vi "read_params.vi"(8 "error in (no error)":errorcluster, 11 "GaussianNB in":refnum<class "GaussianNB.lvclass">) -> (0 "error out":errorcluster, 2 "params":T1={"priors"=[], "var_smoothing"=1e-09}, 3 "GaussianNB out":refnum<class "GaussianNB.lvclass">)   [LabVIEW 2020, in "GaussianNB.lvclass"]
uses:
  GaussianNB.lvclass
  Controls/gaussian_nb_params.ctl
  GaussianNB.lvclass/GaussianNB.ctl
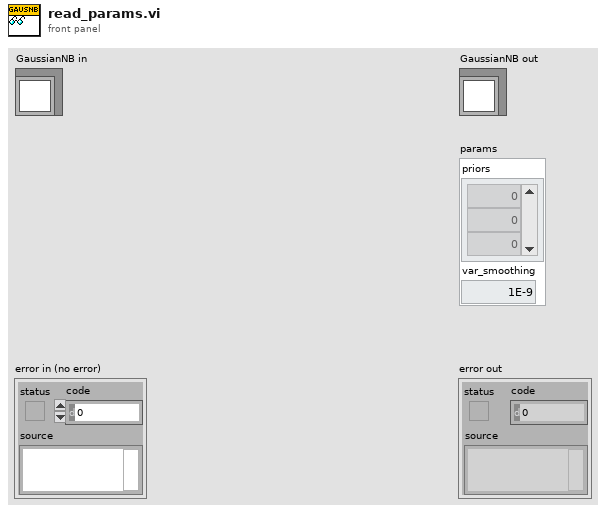
[diagram p1: front panel]
types:
  T1 = typedef "gaussian_nb_params.ctl" = cluster{"priors":dbl[], "var_smoothing":dbl}
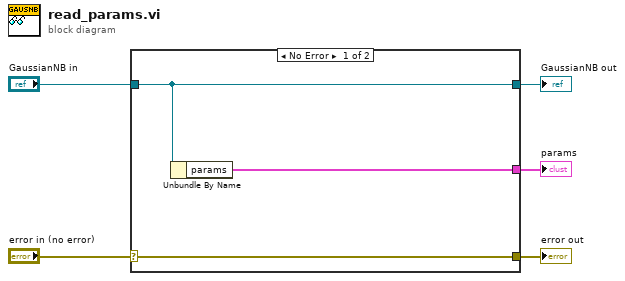
[diagram p0: block diagram]
diagram:
  n1 = case shown="No Error" "error in (no error)" {
    selector: "error in (no error)" -> [w8 w9]
    tunnel: [w8 w9] -> w4
    tunnel: [w7 w10] -> w2
    tunnel: "GaussianNB in" -> [w7 w10]
    tunnel: [w6 _] -> w1
    frame No Error {
      n2 = Unbundle By Name(w7) -> ("params"=w6:T1)
    }
    frame Error {
    }
  }
  "error out" <- w4
  "GaussianNB out" <- w2
  "params" <- w1
